vi "Sequence.FormatChannelName.vi"(10 "ScaleUnits":string, 11 "Name":string) -> (3 "ChannelName":string)   [LabVIEW 2015, in "Single Station Execution.lvlib"]
uses:
  Single Station Execution.lvlib
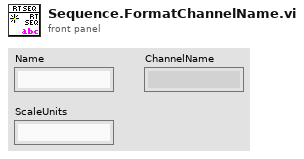
[diagram p1: front panel]
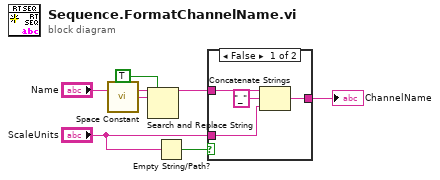
[diagram p0: block diagram]
diagram:
  n1 = call <vilib>:"Space Constant.vi"() -> ("String"=w4:string)
  n2 = Search and Replace String(replace all?=TRUE ("replace all? (F)"), input string="Name", search string=w4) -> (result string=w6:string)  [unwired: 5 in, 3 out]
  n3 = Empty String/Path?(string/path="ScaleUnits") -> (empty?=w1:bool)
  n4 = case shown="False" w1 {
    tunnel: [w11 w12] -> w7
    tunnel: w6 -> [w9 w12]
    tunnel: "ScaleUnits" -> [w8 _]
    frame False {
      n5 = Concatenate Strings(w9, "_" ("string"), w8) -> (w11:string)
    }
    frame True {
    }
  }
  "ChannelName" <- w7
